vi "takeIMAGE_S.vi"(0 "Camera Name":refnum<k21>="cam0" caption="IMAQdx Session") -> (1 "Current image":T1(plugin-control), 2 "error in (no error)":errorcluster)   [LabVIEW 2019]
doc: "Takes one picture (edit block diagram to change) and store in a buffer to be processed"
uses:
  <vilib>/vision/driver/IMAQdx.llb/IMAQdx Acquisition Mode.ctl
  <vilib>/vision/driver/IMAQdx.llb/IMAQdx Buffer Number Mode.ctl
  <vilib>/vision/driver/NI_Vision_Acquisition_Software.lvlib
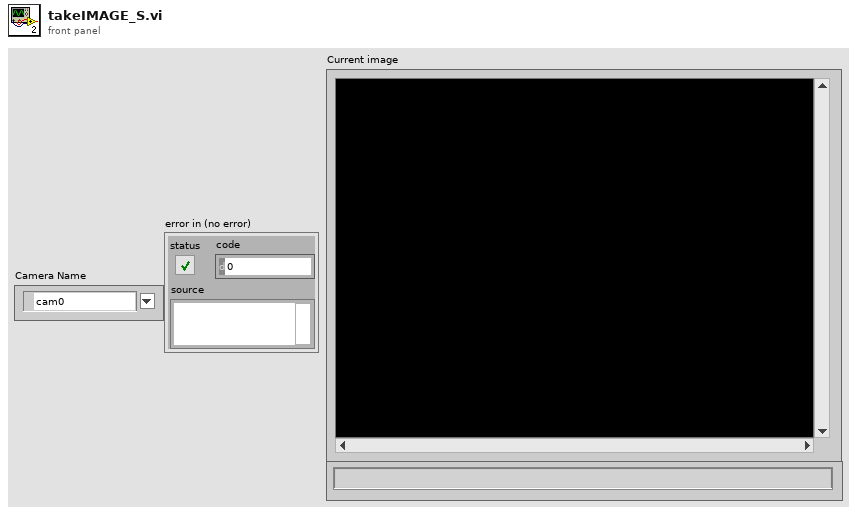
[diagram p1: front panel]
types:
  T1 = typedef "IMAQ Image.ctl" = refnum<image>
  T2 = typedef "NI_Vision_Acquisition_Software.lvlib/IMAQdx Buffer Number Mode.ctl" = enum32{"Next", "Last", "Buffer Number", "Every", "Last New"}
  T3 = typedef "NI_Vision_Acquisition_Software.lvlib/IMAQdx Acquisition Mode.ctl" = enum32{"One Shot", "Continuous"}
  T4 = typedef "IMAQdx.ctl" = refnum<k21>
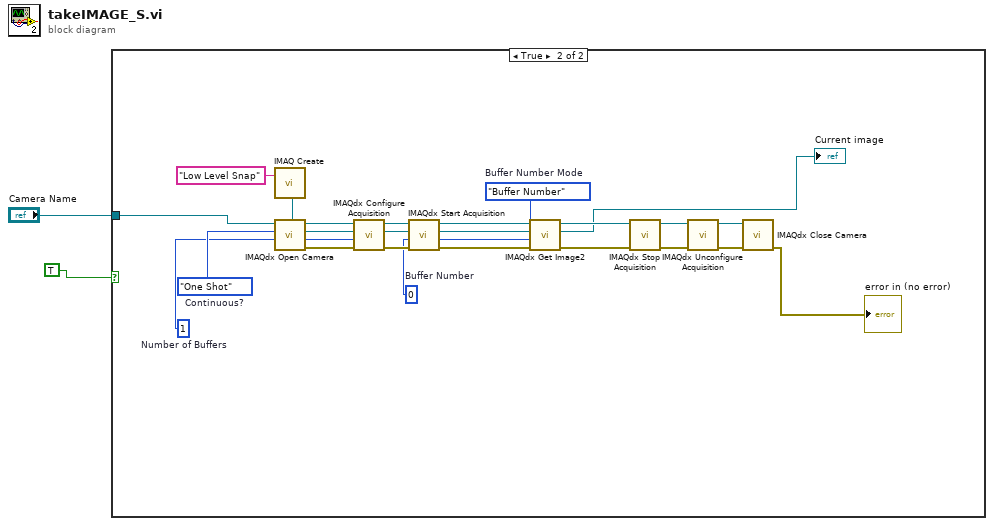
[diagram p0: block diagram]
diagram:
  n1 = case shown="True" TRUE {
    tunnel: "Camera Name" -> [_ w22]
    frame False {
    }
    frame True {
      w6 = u32 0  # Buffer Number
      w13 = IMAQdx_Buffer_Number_Mode."Buffer Number"  # Buffer Number Mode
      w14 = u32 1  # Number of Buffers
      w15 = IMAQdx_Acquisition_Mode."One Shot"  # Continuous?
      n2 = call "IMAQ Create"("Image Name"="Low Level Snap") -> ("New Image"=w23:T1)  [unwired: 3 in, 2 out]
      n3 = call <vilib>:"IMAQdx Open Camera.vi"("Session In"=w22) -> ("error out"=w18:errorcluster, "Session Out"=w20:T4)  [unwired: 2 in, 7 out]
      n4 = call <vilib>:"IMAQdx Configure Acquisition.vi"("error in"=w18, "Number of Buffers"=w14, "Continuous?"=w15, "Session In"=w20) -> ("error out"=w21:errorcluster, "Session Out"=w19:T4)  [unwired: 6 out]
      n5 = call <vilib>:"IMAQdx Start Acquisition.vi"("error in"=w21, "Session In"=w19) -> ("error out"=w17:errorcluster, "Session Out"=w16:T4)  [unwired: 8 out]
      n6 = call <vilib>:"IMAQdx Get Image2.vi"("Buffer Number Mode (Next)"=w13, "error in"=w17, "Buffer Number In"=w6, "Image In"=w23, "Session In"=w16) -> ("error out"=w10:errorcluster, "Image Out"=→"Current image":T1, "Session Out"=w7:T4)  [unwired: 3 in, 1 out]
      n7 = call <vilib>:"IMAQdx Stop Acquisition.vi"("error in"=w10, "Session In"=w7) -> ("error out"=w11:errorcluster, "Session Out"=w12:T4)  [unwired: 8 out]
      n8 = call <vilib>:"IMAQdx Unconfigure Acquisition.vi"("error in"=w11, "Session In"=w12) -> ("error out"=w9:errorcluster, "Session Out"=w8:T4)  [unwired: 8 out]
      n9 = call <vilib>:"IMAQdx Close Camera.vi"("error in"=w9, "Session In"=w8) -> ("error out"=→"error in (no error)":errorcluster)  [unwired: 9 out]
    }
  }
